vi "4-3.vi"() -> ()   [LabVIEW 2017]
panel:
  out "sqrt（x）":ext format="%_5f"
  in  "x":i32
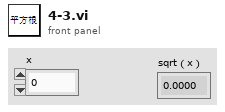
[diagram p1: front panel]
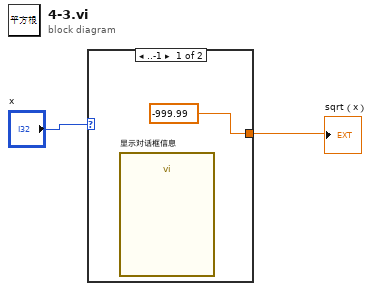
[diagram p0: block diagram]
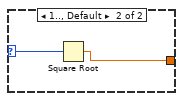
[diagram p2: hidden frame]
diagram:
  n1 = case shown="..-1" "x" {
    selector: "x" -> [_ w5]
    tunnel: [-999.99 ("数值") w4] -> w1
    frame ..-1 {
      n2 = call "显示对话框信息"() -> ()  [unwired: 10 in, 2 out]
    }
    frame 1.., Default {
      n3 = Square Root(x=w5) -> (sqrt(x)=w4:dbl)
    }
  }
  "sqrt（x）" <- w1
